vi "GVSDataView Pane Resize Proc.vi"(8 "DataView Index":i32, 11 "VI Ref":refnum<vi>) -> ()   [LabVIEW 2013]
uses:
  GVSNew View Global.vi
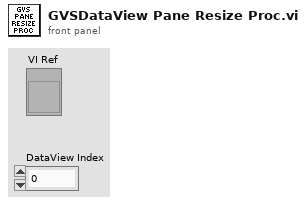
[diagram p1: front panel]
types:
  T1 = typedef "Graph Main Info Cluster.ctl" = cluster{"Selected_BarIdx":i32, "Selected_PanelIdx":i32, "Graph Main VIRef":refnum<vi>, "ToolBarClick":bool, "Spliter Ref Array":refnum<vi>[], "Panel Ref Array":refnum<vi>[], "Spliter_matrix":i32[][], "Panel_matrix":i32[][], "child_spliterIdx_matrix":i32[][], "split_pos_matrix":i32[][], "Title State":bool, "sQueueName":string, "Frame nID":i32, "Graph VIRef Array":cluster{"Graph VIRef":refnum<vi>, "Panel Idx":i32, "Frame VIRef":refnum<vi>, "Icon Ring":i32, "Graph Type":string}[], "View Type":string}
  T2 = typedef "LVRectTypeDef.ctl" = cluster{"Left":i16, "Top":i16, "Right":i16, "Bottom":i16}
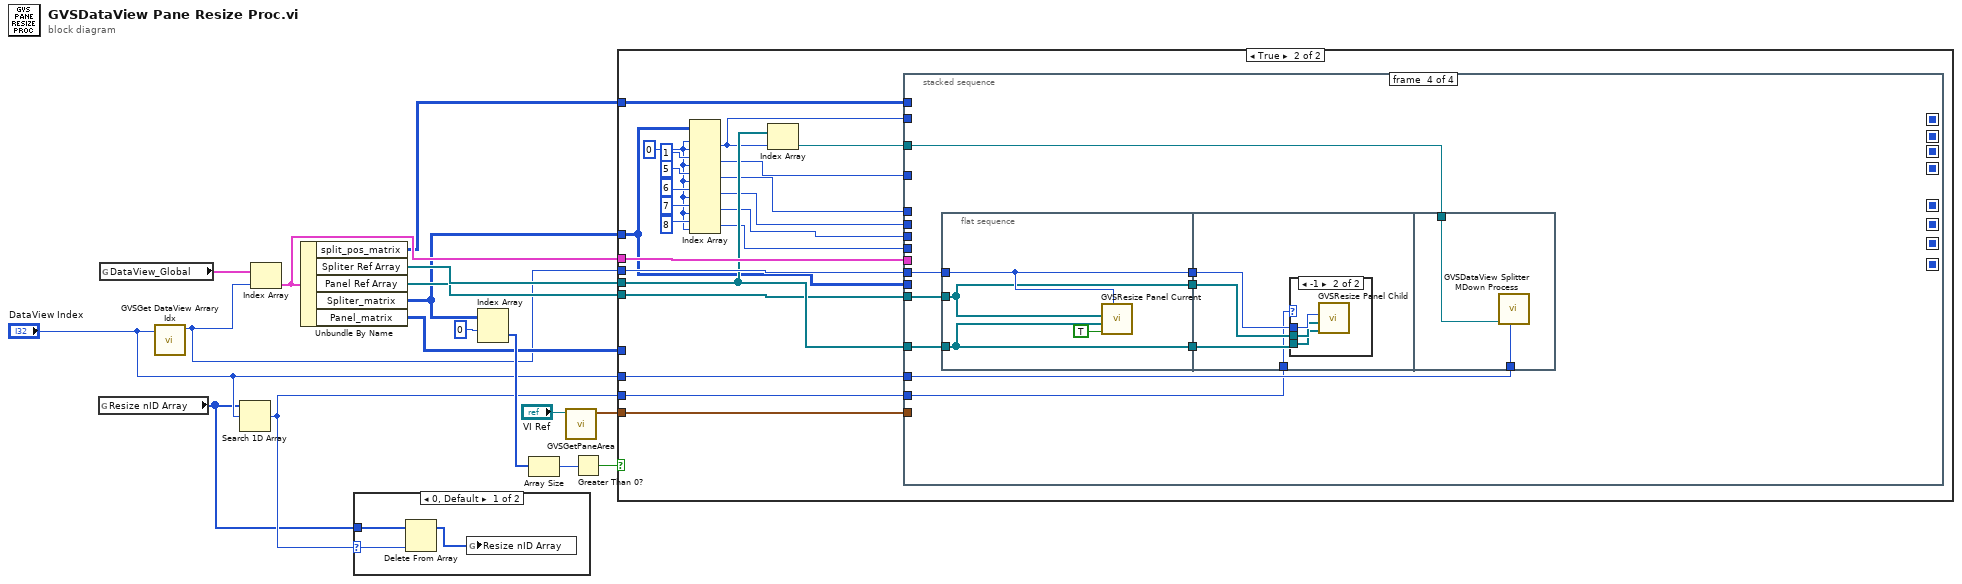
[diagram p0: block diagram]
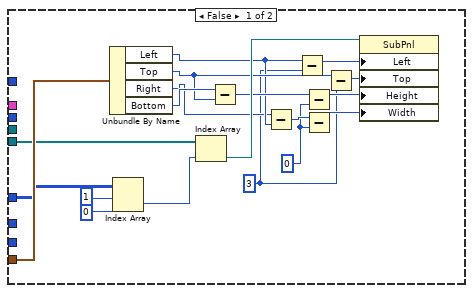
[diagram p3: hidden frame]
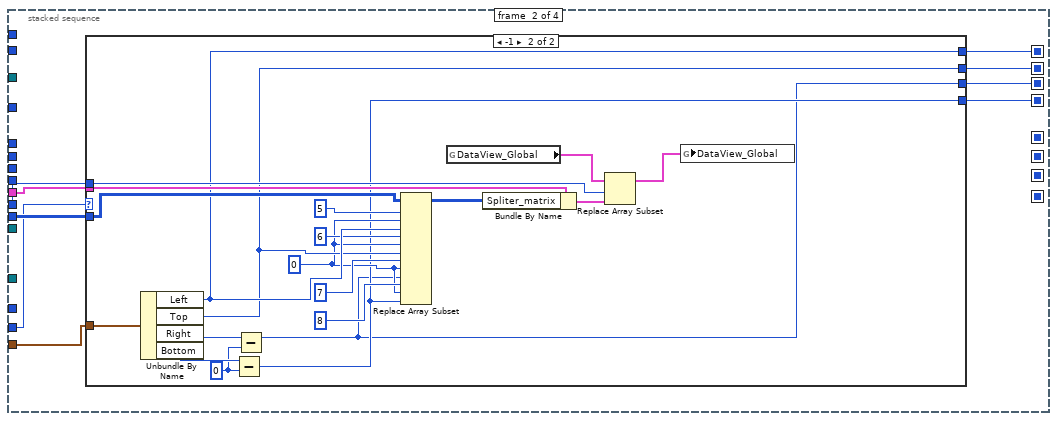
[diagram p5: hidden frame]
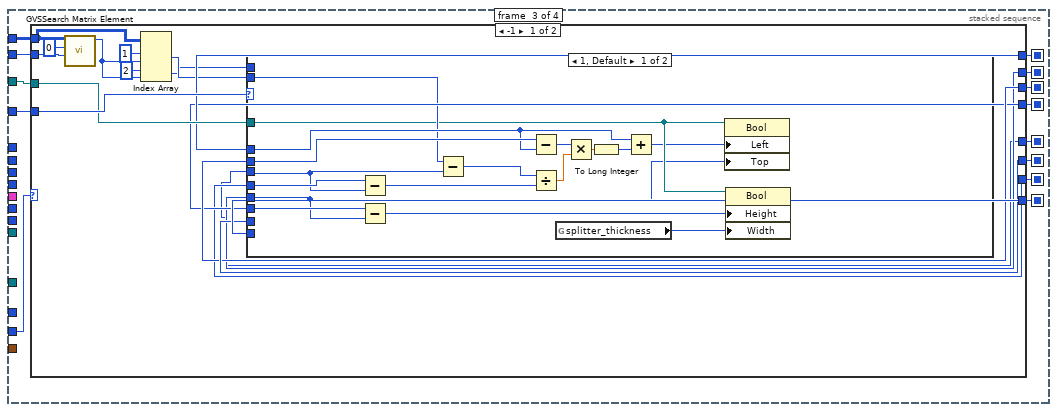
[diagram p7: hidden frame]
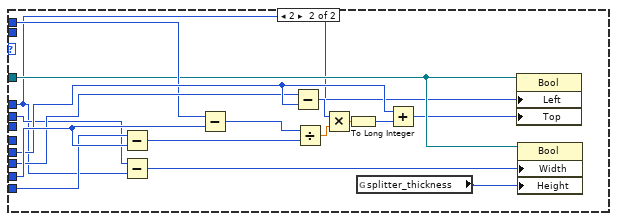
[diagram p8: hidden frame]
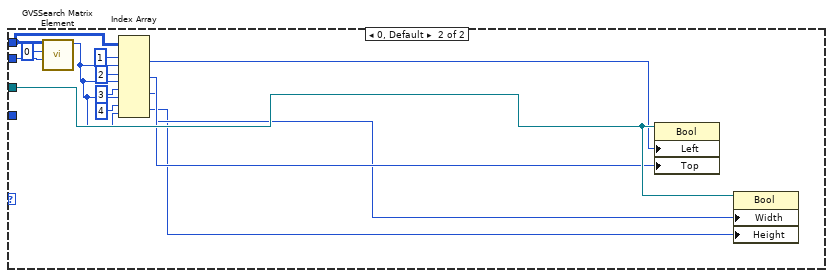
[diagram p9: hidden frame]
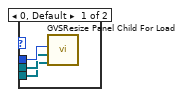
[diagram p10: hidden frame]
diagram:
  n1 = global read "GVSNew View Global.vi" "Resize nID Array"() -> (w1:i32[])
  n2 = global read "GVSNew View Global.vi" "DataView_Global"() -> (w12:T1[])
  n3 = call "GVSGet DataView Arrary Idx.vi"("DataView Idx In"="DataView Index") -> ("DataView Arrary Idx out"=w5:i32)  [unwired: 10 in]
  n4 = Search 1D Array(1D array=w1, element="DataView Index") -> (index of element=w2:i32)  [unwired: 1 in]
  n5 = Index Array(array=w12, index=w5) -> (element=w13:T1)
  n6 = Unbundle By Name(w13) -> ("split_pos_matrix"=w4:i32[][], "Spliter Ref Array"=w10:refnum<vi>[], "Panel Ref Array"=w9:refnum<vi>[], "Spliter_matrix"=w6:i32[][], "Panel_matrix"=w7:i32[][])
  n7 = case shown="0, Default" w2 {
    selector: w2 -> [w19 _]
    tunnel: w1 -> [w20 _]
    frame 0, Default {
      n8 = Delete From Array(array=w20, index=w19) -> (array with subset deleted=w18:i32[])  [unwired: 1 in, 1 out]
      n9 = global write "GVSNew View Global.vi" "Resize nID Array"(w18) -> ()
    }
    frame -1 {
    }
  }
  n10 = Index Array(array=w6, index (row)=0) -> (element=w16:i32[])  [unwired: 1 in]
  n11 = Array Size(array=w16) -> (size(s)=w15:i32)
  n12 = call "GVSGetPaneArea.vi"("vi reference"="VI Ref") -> ("Content Area Rect"=w11:T2)  [unwired: 10 in]
  n13 = Greater Than 0?(x=w15) -> (x > 0?=w14:bool)
  n14 = case shown="True" w14 {
    tunnel: w6 -> [_ w49]
    tunnel: w10 -> [_ w58]
    tunnel: w13 -> [_ w60]
    tunnel: w5 -> [_ w59]
    tunnel: w9 -> [w38 w57]
    tunnel: w11 -> [w39 w56]
    tunnel: w7 -> [w30 _]
    tunnel: "DataView Index" -> [_ w45]
    tunnel: w4 -> [_ w42]
    tunnel: w2 -> [_ w40]
    frame False {
      w21 = 3
      w24 = i16 0 ("y")
      n15 = Unbundle By Name(w39) -> ("Left"=w32:i16, "Top"=w35:i16, "Right"=w31:i16, "Bottom"=w36:i16)
      n16 = Index Array(array=w30, index (row)=1, index (col)=0) -> (element=w27:i32)
      n17 = Index Array(array=w38, index=w27) -> (element=w37:refnum<vi>)
      n18 = Subtract(x=w36, y=w35) -> (x-y=w34:i16)
      n19 = Subtract(x=w31, y=w32) -> (x-y=w33:i16)
      n20 = Subtract(x=w32, y=w21) -> (x-y=w23:i32)
      n21 = Subtract(x=w34, y=w24) -> (x-y=w25:i16)
      n22 = Subtract(x=w33, y=w24) -> (x-y=w26:i16)
      n23 = Subtract(x=w35, y=w21) -> (x-y=w22:i32)
      n24 = property class="SubPnl"(reference=w37, "Left"=w23, "Top"=w22, "Height"=w25, "Width"=w26) -> ()  [unwired: 1 in, 2 out]
    }
    frame True {
      w50 = 0 ("disabled index (col)")
      n25 = Index Array(array=w49, index (row) #1=w50, index (col) #1=w50, index (row) #2=1 ("index (row)"), index (col) #2=w50, index (row) #3=5 ("index (row)"), index (col) #3=w50, index (row) #4=6 ("index (row)"), index (col) #4=w50, index (row) #5=7 ("index (row)"), index (col) #5=w50, index (row) #6=8 ("index (row)"), index (col) #6=w50) -> (element #1=w41:i32, element #2=w48:i32, element #3=w47:i32, element #4=w46:i32, element #5=w44:i32, element #6=w43:i32)
      n26 = Index Array(array=w58, index=w41) -> (element=w61:refnum<vi>)
      n27 = stacked-sequence {
        seq-local: [w62 _ _ _] -> [_ _ w105 _]
        seq-local: [w63 _ _ _] -> [_ _ w99 _]
        seq-local: [w64 _ _ _] -> [_ _ w104 _]
        seq-local: [w65 _ _ _] -> [_ _ w98 _]
        seq-local: [_ w70 _ _] -> [_ _ w102 _]
        seq-local: [_ w69 _ _] -> [_ _ w100 _]
        seq-local: [_ w67 _ _] -> [_ _ w103 _]
        seq-local: [_ w68 _ _] -> [_ _ w101 _]
        tunnel: w61 -> [_ _ w106 w175]
        tunnel: w60 -> [_ w74 _ _]
        tunnel: w49 -> [_ w71 _ _]
        tunnel: w59 -> [_ w73 _ w176]
        tunnel: w48 -> [_ _ w107 _]
        tunnel: w47 -> [w65 _ _ _]
        tunnel: w46 -> [w64 _ _ _]
        tunnel: w44 -> [w63 _ _ _]
        tunnel: w43 -> [w62 _ _ _]
        tunnel: w58 -> [_ _ _ w178]
        tunnel: w57 -> [_ _ _ w177]
        tunnel: w56 -> [_ w72 _ _]
        tunnel: w45 -> [_ _ _ w174]
        tunnel: w42 -> [_ _ w96 _]
        tunnel: w41 -> [_ _ w97 _]
        tunnel: w40 -> [_ w66 w95 w173]
        frame #0 {
        }
        frame #1 {
          n28 = case shown="-1" w66 {
            tunnel: w74 -> [_ w94]
            tunnel: w73 -> [_ w92]
            tunnel: w72 -> [_ w89]
            tunnel: w71 -> [_ w88]
            tunnel: [_ w86] -> w70
            tunnel: [_ w84] -> w69
            tunnel: [_ w78] -> w68
            tunnel: [_ w76] -> w67
            frame 0, Default {
            }
            frame -1 {
              w75 = i16 0 ("y")
              w80 = 0 ("index (col)")
              n29 = Unbundle By Name(w89) -> ("Left"=w86:i16, "Top"=w84:i16, "Right"=w82:i16, "Bottom"=w77:i16)
              n30 = Subtract(x=w77, y=w75) -> (x-y=w78:i16)
              n31 = Subtract(x=w82, y=w75) -> (x-y=w76:i16)
              n32 = Replace Array Subset(array=w88, new element #1=w86, index (row) #1=5 ("disabled index (row)"), index (col) #1=w80, new element #2=w84, index (row) #2=6 ("disabled index (row)"), index (col) #2=w80, new element #3=w76, index (row) #3=7 ("disabled index (row)"), index (col) #3=w80, new element #4=w78, index (row) #4=8 ("disabled index (row)"), index (col) #4=w80) -> (w79:i32[][])
              n33 = global read "GVSNew View Global.vi" "DataView_Global"() -> (w90:T1[])
              n34 = Bundle By Name(cluster=w94, "Spliter_matrix"=w79) -> (w93:T1)
              n35 = Replace Array Subset(array=w90, new element=w93, index=w92) -> (w91:T1[])
              n36 = global write "GVSNew View Global.vi" "DataView_Global"(w91) -> ()
            }
          }
        }
        frame #2 {
          n37 = case shown="-1" w95 {
            tunnel: w107 -> [w125 _]
            tunnel: w106 -> [w124 w167]
            tunnel: w105 -> [w123 _]
            tunnel: w104 -> [w122 _]
            tunnel: w103 -> [w121 _]
            tunnel: w102 -> [w120 _]
            tunnel: w101 -> [w119 _]
            tunnel: w100 -> [w118 _]
            tunnel: w99 -> [w117 _]
            tunnel: w98 -> [w116 _]
            tunnel: w97 -> [w115 w172]
            tunnel: w96 -> [w113 w170]
            frame -1 {
              n38 = call "GVSSearch Matrix Element.vi"("element"=w115, "index (row)"=0, "matrix in"=w113) -> ("index of element"=w110:i32)  [unwired: 8 in]
              n39 = Index Array(array=w113, index (row) #1=1 ("disabled index (row)"), index (col) #1=w110, index (row) #2=2 ("disabled index (row)"), index (col) #2=w110) -> (element #1=w111:i32, element #2=w108:i32)
              n40 = case shown="1, Default" w125 {
                tunnel: w124 -> [w131 w147]
                tunnel: w117 -> [w142 _]
                tunnel: w123 -> [_ w151]
                tunnel: w122 -> [_ w154]
                tunnel: w121 -> [w136 w150]
                tunnel: w120 -> [w135 w146]
                tunnel: w119 -> [w134 w152]
                tunnel: w118 -> [w128 w153]
                tunnel: w116 -> [w133 _]
                tunnel: w111 -> [w132 _]
                tunnel: w108 -> [_ w149]
                frame 1, Default {
                  n41 = Subtract(x=w142, y=w133) -> (x-y=w141:i32)
                  n42 = Subtract(x=w134, y=w128) -> (x-y=w127:i16)
                  n43 = Subtract(x=w132, y=w133) -> (x-y=w140:i32)
                  n44 = Subtract(x=w136, y=w135) -> (x-y=w137:i16)
                  n45 = Divide(x=w140, y=w141) -> (x/y=w139:dbl)
                  n46 = global read "GVSNew View Global.vi" "splitter_thickness"() -> (w126:u32)
                  n47 = Multiply(x=w137, y=w139) -> (x*y=w138:dbl)
                  n48 = To Long Integer(number=w138) -> (32bit integer=w130:i32)
                  n49 = Add(x=w135, y=w130) -> (x+y=w129:i32)
                  n50 = property class="Bool"(reference=w131, "Left"=w129, "Top"=w128) -> ()  [unwired: 1 in, 2 out]
                  n51 = property class="Bool"(reference=w131, "Height"=w127, "Width"=w126) -> ()  [unwired: 1 in, 2 out]
                }
                frame 2 {
                  n52 = Subtract(x=w151, y=w154) -> (x-y=w159:i32)
                  n53 = Subtract(x=w150, y=w146) -> (x-y=w144:i16)
                  n54 = Subtract(x=w149, y=w154) -> (x-y=w158:i32)
                  n55 = Subtract(x=w152, y=w153) -> (x-y=w155:i16)
                  n56 = Divide(x=w158, y=w159) -> (x/y=w157:dbl)
                  n57 = Multiply(x=w155, y=w157) -> (x*y=w156:dbl)
                  n58 = To Long Integer(number=w156) -> (32bit integer=w148:i32)
                  n59 = global read "GVSNew View Global.vi" "splitter_thickness"() -> (w143:u32)
                  n60 = Add(x=w153, y=w148) -> (x+y=w145:i32)
                  n61 = property class="Bool"(reference=w147, "Left"=w146, "Top"=w145) -> ()  [unwired: 1 in, 2 out]
                  n62 = property class="Bool"(reference=w147, "Width"=w144, "Height"=w143) -> ()  [unwired: 1 in, 2 out]
                }
              }
            }
            frame 0, Default {
              n63 = call "GVSSearch Matrix Element.vi"("element"=w172, "index (row)"=0, "matrix in"=w170) -> ("index of element"=w164:i32)  [unwired: 8 in]
              n64 = Index Array(array=w170, index (row) #1=1 ("disabled index (row)"), index (col) #1=w164, index (row) #2=2 ("disabled index (row)"), index (col) #2=w164, index (row) #3=3 ("disabled index (row)"), index (col) #3=w164, index (row) #4=4 ("disabled index (row)"), index (col) #4=w164) -> (element #1=w163:i32, element #2=w162:i32, element #3=w161:i32, element #4=w160:i32)
              n65 = property class="Bool"(reference=w167, "Left"=w163, "Top"=w162) -> ()  [unwired: 1 in, 2 out]
              n66 = property class="Bool"(reference=w167, "Width"=w161, "Height"=w160) -> ()  [unwired: 1 in, 2 out]
            }
          }
        }
        frame #3 {
          n67 = flat-sequence {
            tunnel: [w184] -> w181
            tunnel: [w183] -> w180
            tunnel: [w182] -> w179
            tunnel: w177 -> [w183]
            tunnel: w178 -> [w182]
            tunnel: w176 -> [w184]
            tunnel: w181 -> [w189]
            tunnel: w180 -> [w188]
            tunnel: w179 -> [w187]
            tunnel: w173 -> [w186]
            tunnel: w175 -> [w197]
            tunnel: w174 -> [w196]
            frame #0 {
              n68 = call "GVSResize Panel Current.vi"("DataView Array Idx"=w184, "close_panel"=TRUE, "spliter array"=w182, "SubPanel array"=w183) -> ()  [unwired: 8 in]
            }
            frame #1 {
              n69 = case shown="-1" w186 {
                tunnel: w189 -> [w192 w195]
                tunnel: w188 -> [w191 w194]
                tunnel: w187 -> [w190 w193]
                frame 0, Default {
                  n70 = call "GVSResize Panel Child For Load.vi"("spliter array"=w190, "SubPanel array"=w191, "DataView Array Idx"=w192) -> ()  [unwired: 9 in]
                }
                frame -1 {
                  n71 = call "GVSResize Panel Child.vi"("spliter array"=w193, "SubPanel array"=w194, "DataView Array Idx"=w195) -> ()  [unwired: 9 in]
                }
              }
            }
            frame #2 {
              n72 = call "GVSDataView Splitter MDown Process.vi"("DataView Index"=w196, "Selected Spliter Ref"=w197) -> ()  [unwired: 9 in, 1 out]
            }
          }
        }
      }
    }
  }
